vi "ReducePixMapForThumbnail.vi"(9 "New Width":i32=120, 10 "New Height":i32=120, 11 "path to PNG file":path) -> (3 "new picture":picture)   [LabVIEW 2024, in "Application.lvclass"]
uses:
  Application.lvclass
  <vilib>/picture/picture.llb/Draw True-Color Pixmap.vi
  Application.lvclass/Application.ctl
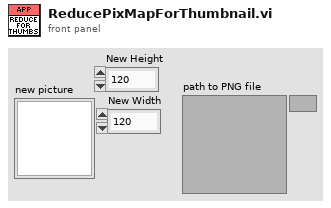
[diagram p1: front panel]
types:
  T1 = typedef "imagedata.ctl" = cluster{"image type":i32, "image depth":i32, "image":u8[], "mask":u8[], "colors":u32[], "Rectangle":cluster{"left":i16, "top":i16, "right":i16, "bottom":i16}}
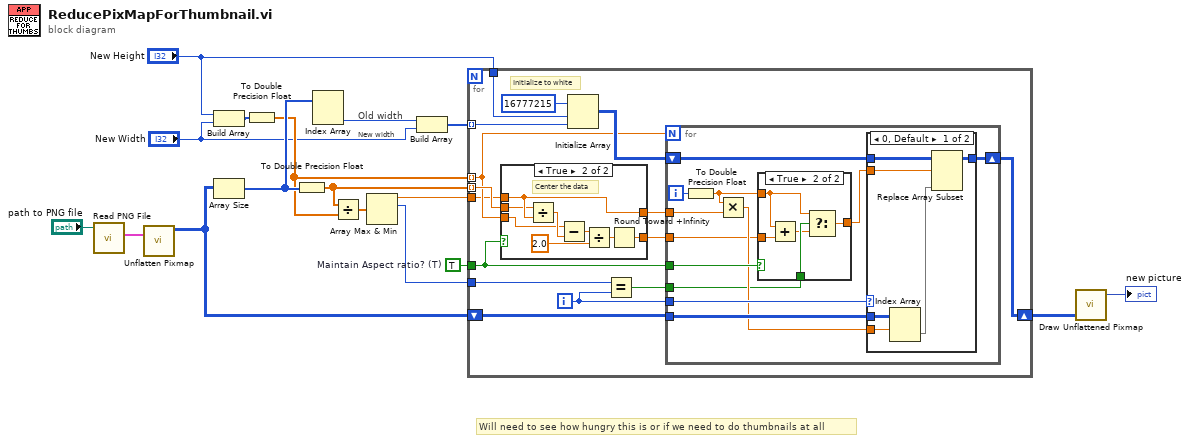
[diagram p0: block diagram]
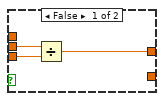
[diagram p2: hidden frame]
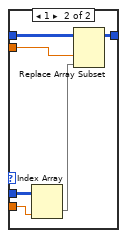
[diagram p4: hidden frame]
diagram:
  w12 = TRUE  # Maintain Aspect ratio? (T)
  # "Will need to see how hungry this is or if we need to do thumbnails at all"
  # "New width"
  # "Old width"
  n1 = call <vilib>:"Read PNG File.vi"("path to PNG file"="path to PNG file") -> ("image data"=w5:T1)  [unwired: 8 in, 2 out]
  n2 = call <vilib>:"Unflatten Pixmap.vi"("image data"=w5) -> ("24-bit pixmap"=w4:u32[][])  [unwired: 4 in, 6 out]
  n3 = Build Array("New Height", "New Width") -> (w10:i32[])
  n4 = Array Size(array=w4) -> (size(s)=w16:i32[])
  n5 = To Double Precision Float(number=w10) -> (double precision float=w14:dbl[])
  n6 = To Double Precision Float(number=w16) -> (double precision float=w15:dbl[])
  n7 = Index Array(array=w16) -> (element #2=w6:i32)  [unwired: 2 in, 1 out]
  n8 = Divide(x=w15, y=w14) -> (x/y=w7:dbl[])
  n9 = Array Max & Min(array=w7) -> (max value=w11:dbl, max index (indices)=w13:i32)  [unwired: 2 out]
  n10 = Build Array(w6, "New Width") -> (w9:i32[])
  n11 = for {
    tunnel: w15 -> [w26] mode=indexing
    tunnel: w14 -> [w24] mode=indexing
    shift-right: [w32] -> w8
    shift-left: w4 -> [w31]
    tunnel: "New Height" -> [w28]
    tunnel: w9 -> [w27] mode=indexing
    tunnel: w11 -> [w23]
    tunnel: w12 -> [w18]
    tunnel: w13 -> [w20]
    i -> [w21]
    # "Initialize to white"
    n12 = case shown="True" w18 {
      tunnel: w26 -> [w35 w37]
      tunnel: [w34 w43] -> w25
      tunnel: w24 -> [w33 w36]
      tunnel: w23 -> [_ w43]
      tunnel: [_ w38] -> w22
      frame False {
        n13 = Divide(x=w35, y=w33) -> (x/y=w34:dbl)
      }
      frame True {
        # "Center the data"
        n14 = Divide(x=w37, y=w43) -> (x/y=w39:dbl)
        n15 = Subtract(x=w36, y=w39) -> (x-y=w40:dbl)
        n16 = Divide(x=w40, y=2.0) -> (x/y=w42:dbl)
        n17 = Round Toward +Infinity(x=w42) -> (ceil(x): smallest int >= x=w38:dbl)
      }
    }
    n18 = Initialize Array(u32 16777215, w28, w27) -> (w29:u32[][])
    n19 = Equal?(x=w20, y=w21) -> (x = y?=w19:bool)
    n20 = for {
      N: w24 -> [_]
      tunnel: w25 -> [w55]
      tunnel: w31 -> [w54]
      shift-right: [w51] -> w32
      shift-left: w29 -> [w52]
      tunnel: w21 -> [w53]
      tunnel: w18 -> [w50]
      tunnel: w22 -> [w45]
      tunnel: w19 -> [w46]
      i -> [w47]
      n21 = To Double Precision Float(number=w47) -> (double precision float=w44:dbl)
      n22 = Multiply(x=w44, y=w55) -> (x*y=w49:dbl)
      n23 = case shown="True" w50 {
        tunnel: [w56 w61] -> w48
        tunnel: w44 -> [w56 w59]
        tunnel: w46 -> [_ w60]
        tunnel: w45 -> [_ w57]
        frame False {
        }
        frame True {
          n24 = Add(x=w59, y=w57) -> (x+y=w58:dbl)
          n25 = Select(t=w59, s=w60, f=w58) -> (s? t:f=w61:dbl)
        }
      }
      n26 = case shown="0, Default" w53 {
        tunnel: w54 -> [w67 w73]
        tunnel: w49 -> [w63 w69]
        tunnel: w52 -> [w66 w72]
        tunnel: [w65 w71] -> w51
        tunnel: w48 -> [w62 w68]
        frame 0, Default {
          n27 = Index Array(array=w67, index (row)=w63) -> (element=w64:u32[])  [unwired: 1 in]
          n28 = Replace Array Subset(array=w66, new element=w64, index (row)=w62) -> (w65:u32[][])  [unwired: 1 in]
        }
        frame 1 {
          n29 = Index Array(array=w73, index (col)=w69) -> (element=w70:u32[])  [unwired: 1 in]
          n30 = Replace Array Subset(array=w72, new element=w70, index (col)=w68) -> (w71:u32[][])  [unwired: 1 in]
        }
      }
    }
  }
  n31 = call-poly <vilib>:"Draw Unflattened Pixmap.vi"("data (RGB format)"=w8) -> ("new picture"=→"new picture":picture)  [unwired: 8 in]
